vi "Process DeviceID Array.vi"(8 "error in":errorcluster, 11 "DeviceID Array":T1[](array[typedef])) -> (0 "error out":errorcluster, 3 "Array":T1[][](array[typedef]))   [LabVIEW 2018, in "EMS User Interface Actor.lvlib" / "EMS User Interface.lvclass"]
uses:
  EMS User Interface.lvclass
  <vilib>/ORNL/CSEISMIC DDS/CSEISMIC DDS Base/Data Types/Controls/DeviceClass Selector.ctl
  <vilib>/ORNL/CSEISMIC DDS/CSEISMIC DDS Base/Data Types/Controls/DeviceID.ctl
  <vilib>/ORNL/CSEISMIC DDS/CSEISMIC DDS Base/CSEISMIC DDS.lvclass
panel:
  in  "DeviceClass":T2 format="%04x" items=["Invalid"=0, "IED"=256, "DER"=512, "Relay"=768, "Meter"=1024, "Load"=1280, "Forecast"=1536, "Price"=1792, "Energy Storage"=513, "PV"=514, "Generator"=515, "Smart Relay"=769, "PCC"=770, "Smart Meter"=1025, "PMU"=1026, "HVAC"=1281]
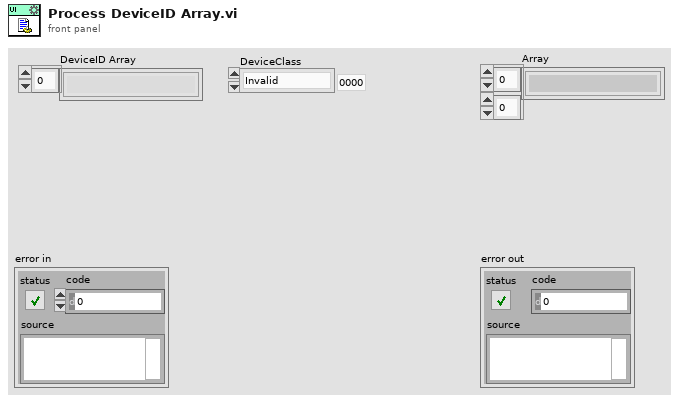
[diagram p1: front panel]
types:
  T1 = typedef "CSEISMIC DDS.lvlib/CSEISMIC DDS.lvclass/DeviceID.ctl" = string
  T2 = typedef "CSEISMIC DDS.lvlib/CSEISMIC DDS.lvclass/DeviceClass Selector.ctl" = u16
  T3 = typedef "LVStringsAndValuesArrayTypeDef.ctl" = cluster{"String":string, "Value":ext}[]
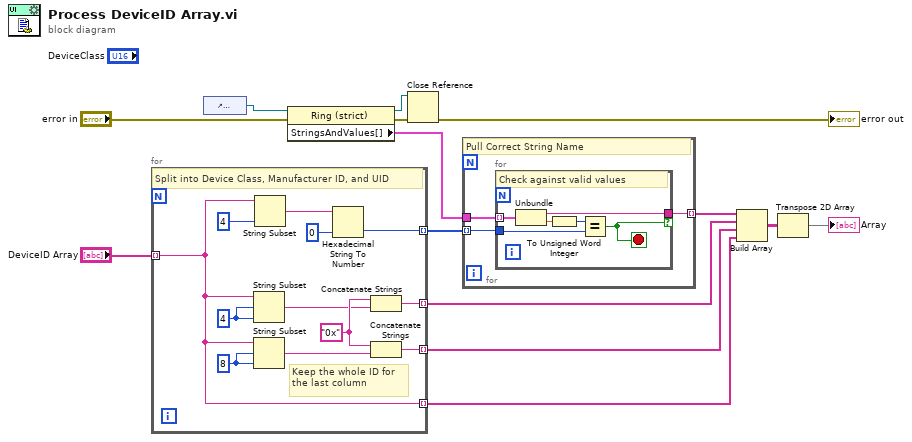
[diagram p0: block diagram]
diagram:
  n1 = for {
    tunnel: "DeviceID Array" -> [w26] mode=indexing
    tunnel: [w19] -> w8 mode=indexing
    tunnel: [w16] -> w2 mode=indexing
    tunnel: [w17] -> w7 mode=indexing
    tunnel: [w26] -> w5 mode=indexing
    w21 = "0x" ("string")
    w23 = 8 ("length (rest)")
    w24 = 4 ("length (rest)")
    # "Keep the whole ID for the last column"
    # "Split into Device Class, Manufacturer ID, and UID"
    n2 = String Subset(string=w26, offset (0)=w24, length (rest)=w24) -> (substring=w18:T1)
    n3 = String Subset(string=w26, offset (0)=w23, length (rest)=w23) -> (substring=w20:T1)
    n4 = String Subset(string=w26, length (rest)=4 ("length (rest)")) -> (substring=w22:T1)  [unwired: 1 in]
    n5 = Hexadecimal String To Number(string=w22, default (0uL)=u16 0 ("default (0 U32)")) -> (number=w16:u16)  [unwired: 1 in, 1 out]
    n6 = Concatenate Strings(w21, w18) -> (w17:string)
    n7 = Concatenate Strings(w21, w20) -> (w19:string)
  }
  n8 = control-ref of="DeviceClass"() -> (w1:refnum<vi>)
  n9 = property class="Ring (strict)"(reference=w1, error in="error in") -> (reference out=w10:refnum<vi>, error out=w9:errorcluster, "StringsAndValues[]"=w3:T3)
  n10 = Close Reference(reference=w10, error in (no error)=w9) -> (error out=→"error out":errorcluster)
  n11 = for {
    tunnel: w2 -> [w28] mode=indexing
    tunnel: w3 -> [w29]
    tunnel: [w27] -> w4 mode=indexing
    # "Pull Correct String Name"
    n12 = for {
      tunnel: w29 -> [w35] mode=indexing
      tunnel: w28 -> [w32]
      tunnel: [w31] -> w27 if=w30
      stop <- w30 stop-if-true
      # "Check against valid values"
      n13 = Unbundle(w35) -> ("String"=w31:string, "Value"=w34:ext)
      n14 = To Unsigned Word Integer(number=w34) -> (unsigned 16bit integer=w33:u16)
      n15 = Equal?(x=w33, y=w32) -> (x = y?=w30:bool)
    }
  }
  n16 = Build Array(w4, w7, w8, w5) -> (w6:T1[][])
  n17 = Transpose 2D Array(2D array=w6) -> (transposed array=→"Array":T1[][])
